vi "Check challenge data.vi"(8 "error in (no error)":errorcluster, 10 "Challenge Dict":string, 11 "WampScramAuthenticator in":refnum<class "WampScramAuthenticator.lvclass">) -> (0 "error out":errorcluster, 2 "Challene data":T1, 3 "WampScramAuthenticator out":refnum<class "WampScramAuthenticator.lvclass">)   [LabVIEW 2020, in "wamplv.lvlib" / "WampScramAuthenticator.lvclass"]
uses:
  WampScramAuthenticator.lvclass
  TypeDefs/Challenge data.ctl
  TypeDefs/HMAC parameters.ctl
  4072bdce-a1c0-4c5b-b43a-c4f95c553131.vi
  34350c80-a7c2-4687-8bdd-0f0ed74fb3f0.vi
  89772692-b13a-4ddc-a810-6d89972cd41a.vi
  eb56029f-d48b-4cea-82bc-504b726eeb06.vi
  <vilib>/JDP Science/JSONtext/Find Item.vi
  <vilib>/JDP Science/JSONtext/Next JSON Value.vi
  <vilib>/JDP Science/JSONtext/String Subset.vi
  <vilib>/JDP Science/JSONtext/Parsing/Advance past next JSON Value (inlined COPY).vi
  <vilib>/JDP Science/JSONtext/Parsing/Advance past whitespace.vi
  <vilib>/JDP Science/JSONtext/Parsing/Advance past String.vi
  <vilib>/JDP Science/JSONtext/Parsing/Advance past Number.vi
  <vilib>/JDP Science/JSONtext/Parsing/Advance past Line Ending.vi
  <vilib>/Utility/error.llb/Error Cluster From Error Code.vi
  <vilib>/JDP Science/JSONtext/Parsing/Parse Full Path or Item Name.vi
  <vilib>/JDP Science/JSONtext/Parsing/Advance past Array.vi
  <vilib>/JDP Science/JSONtext/Parsing/Advance past Object.vi
  <vilib>/JDP Science/JSONtext/support/Error Cluster From Code.vi
  <vilib>/JDP Science/JSONtext/Offset/Find Item Locations by Path.vi
  <vilib>/JDP Science/JSONtext/JSON text to Variant.vi
  <vilib>/ErrorRing/Error Ring.xnode
  <vilib>/JDP Science/JSONtext/LVClass Serializer/JSONtext LVClass Serializer.lvclass
  WampScramAuthenticator.lvclass/WampScramAuthenticator.ctl
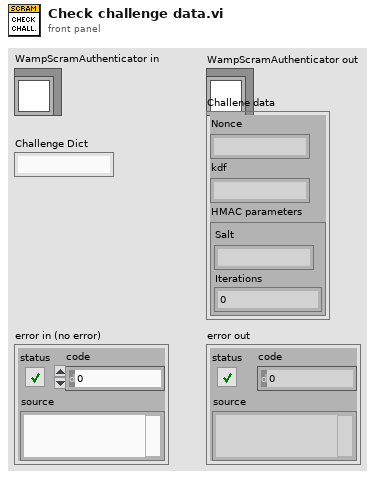
[diagram p1: front panel]
types:
  T1 = typedef "wamplv.lvlib/WampScramAuthenticator.lvclass/Challenge data.ctl" = cluster{"Nonce":string, "kdf":string, "HMAC parameters":T2}
  T2 = typedef "wamplv.lvlib/WampScramAuthenticator.lvclass/HMAC parameters.ctl" = cluster{"Salt":string, "Iterations":i32}
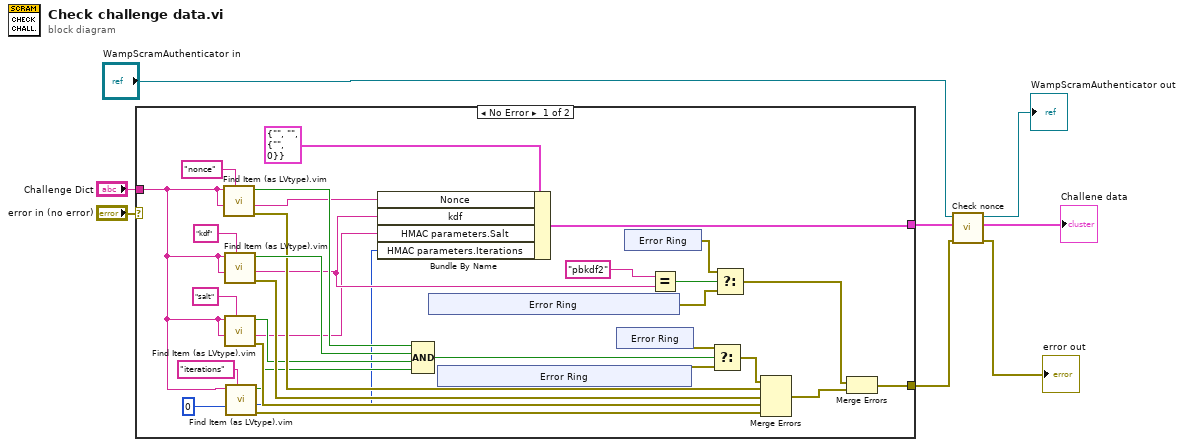
[diagram p0: block diagram]
diagram:
  n1 = case shown="No Error" "error in (no error)" {
    selector: "error in (no error)" -> [_ w50]
    tunnel: "Challenge Dict" -> [w35 _]
    tunnel: [w16 w50] -> w4
    tunnel: [w23 _] -> w1
    frame No Error {
      n2 = call "Find Item (as LVtype).vim"("$Path or Item Name"="nonce", "Data Type and Default Value"=w35, "JSON"=w35) -> ("error out"=w31:errorcluster, "Data"=w25:string, "Found"=w34:bool)  [unwired: 5 in, 1 out]
      n3 = call "Find Item (as LVtype).vim"("$Path or Item Name"="kdf", "Data Type and Default Value"=w35, "JSON"=w35) -> ("error out"=w32:errorcluster, "Data"=w15:string, "Found"=w33:bool)  [unwired: 5 in, 1 out]
      n4 = call "Find Item (as LVtype).vim"("$Path or Item Name"="salt", "Data Type and Default Value"=w35, "JSON"=w35) -> ("error out"=w13:errorcluster, "Data"=w10:string, "Found"=w11:bool)  [unwired: 5 in, 1 out]
      n5 = call "Find Item (as LVtype).vim"("$Path or Item Name"="iterations", "Data Type and Default Value"=0, "JSON"=w35) -> ("error out"=w14:errorcluster, "Data"=w9:i32, "Found"=w12:bool)  [unwired: 5 in, 1 out]
      n6 = Bundle By Name(cluster=T1 {"Nonce"="", "kdf"="", "HMAC parameters"={"Salt"="", "Iterations"=0}} ("Cluster"), "Nonce"=w25, "kdf"=w15, "HMAC parameters.Salt"=w10, "HMAC parameters.Iterations"=w9) -> (w23:T1)
      n7 = Compound Arithmetic op=AND(w34, w33, w11, w12) -> (w30:bool)
      n8 = xnode "Error Ring"() -> ("error out"=w18:errorcluster)
      n9 = xnode "Error Ring"() -> ("error out"=w27:errorcluster)
      n10 = xnode "Error Ring"() -> ("error out"=w29:errorcluster)
      n11 = xnode "Error Ring"() -> ("error out"=w19:errorcluster)
      n12 = Equal?(x="pbkdf2", y=w15) -> (x = y?=w20:bool)
      n13 = Select(t=w29, s=w30, f=w27) -> (s? t:f=w28:errorcluster)
      n14 = Select(t=w19, s=w20, f=w18) -> (s? t:f=w17:errorcluster)
      n15 = Merge Errors(w28, w31, w32, w13, w14) -> (w22:errorcluster)
      n16 = Merge Errors(w17, w22) -> (w16:errorcluster)
    }
    frame Error {
    }
  }
  n17 = call "Check nonce.vi"("error in (no error)"=w4, "Challenge data in"=w1, "WampScramAuthenticator in"="WampScramAuthenticator in") -> ("error out"=→"error out":errorcluster, "Challenge data out"=→"Challene data":T1, "WampScramAuthenticator out"=→"WampScramAuthenticator out":refnum<class "WampScramAuthenticator.lvclass">)  [unwired: 6 in]
